vi "Convert Arc Velocity to Steering Frame Velocity.vi"(11 "arc velocity":T1={"turning radius"=1.0, "tangential velocity"=0.0, "angle from tangent (rad)"=0.0}) -> (3 "steering frame velocity":dbl[](array[numeric]))   [LabVIEW 2017, in "NI_Robotics_Steering Frame.lvclass"]
uses:
  <vilib>/robotics/Steering/Steering Frame/NI_Robotics_Steering Frame.lvclass
  <vilib>/robotics/Steering/Steering Frame/Arc Velocity.ctl
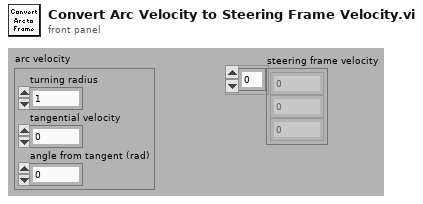
[diagram p1: front panel]
types:
  T1 = typedef "NI_Robotics_Steering Frame.lvclass/Arc Velocity.ctl" = cluster{"turning radius":dbl, "tangential velocity":dbl, "angle from tangent (rad)":dbl}
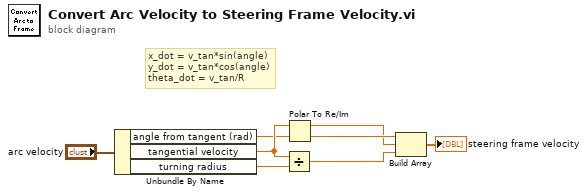
[diagram p0: block diagram]
diagram:
  # "x_dot = v_tan*sin(angle)\ny_dot = v_tan*cos(angle)\ntheta_dot = v_tan/R"
  n1 = Unbundle By Name("arc velocity") -> ("angle from tangent (rad)"=w3:dbl, "tangential velocity"=w4:dbl, "turning radius"=w8:dbl)
  n2 = Divide(x=w4, y=w8) -> (x/y=w7:dbl)
  n3 = Polar To Re/Im(2:w3, 3:w4) -> (0:w2:dbl, 1:w1:dbl)
  n4 = Build Array(w2, w1, w7) -> (→"steering frame velocity":dbl[])
